vi "LoadObserverControlMatrix_zaxis.vi"(8 "NS":u16, 11 "NS_nsw":u16) -> (2 "SS FIFO TimeOut?":bool)   [LabVIEW 2017]
uses:
  fixed-point-ss/typeDefs/Bz_bram.ctl
  fixed-point-ss/typeDefs/Lz_bram.ctl
  fixed-point-ss/typeDefs/Cz_zaxis_bram.ctl
  fixed-point-ss/typeDefs/A_as_vec_bram.ctl
  <vilib>/rvi/interface/RandomDataEmulation/niFpgaRandomDataHandleErrors.vi
  <vilib>/rvi/DataTransferAndStorage/Container/Common/niFpgaContainerExecOnDevCompGetState.vi
  <vilib>/rvi/Emulation/niFpgaEmulationIsFPGAContextNoSignature.vi
  <vilib>/rvi/DataTransferAndStorage/Container/Common/niFpgaContainerGetUniqueNameForEmu.vi
  <vilib>/rvi/Emulation/niFpgaProcessEmulError.vi
  <vilib>/rvi/Emulation/niFpgaSctlEmulationGetInTimedLoop.vi
  <vilib>/rvi/errors/nirviReportUnexpectedCaseInternalError (U32).vi
  <vilib>/rvi/Memory/Memory_Emulation/niFpgaMemoryEmulationCacheClearOnFirstRun.vi
  <vilib>/rvi/Memory/Memory_Emulation/nirvimemoryEmulationManagerCache_MakeExclusive.vi
  <vilib>/rvi/Memory/Memory_Emulation/niFpgaMemoryEmulationValidateCache.vi
  <vilib>/rvi/Memory/Memory_Emulation/nirvimemoryEmulationManagerCache_InsertValue.vi
  <vilib>/Utility/error.llb/Clear Errors.vi
  <vilib>/rvi/Memory/Memory_Emulation/nirvimemoryEmulationManagerCache_ReleaseExclusive.vi
  <vilib>/rvi/Memory/Memory_Emulation/nirvimemoryEmulationManagerCache_GetValue.vi
  <vilib>/rvi/Memory/Memory_Emulation/nirvimemoryEmulationManagerCache_SetValue.vi
  <vilib>/rvi/Emulation/niFpgaSctlEmulationResourceMgr.vi
  <vilib>/rvi/DataTransferAndStorage/Container/XNode/niFpgaContainer.xnode
  <vilib>/rvi/interface/RandomDataEmulation/nirviRandomDataFpgaReadWriteTemplate.vi
  <vilib>/rvi/Memory/Memory_Emulation/niFpgaMemoryEmulationRefIn.vi
panel:
  # "NOTE: Ns is the number of states in the plant. The number of states in the \nobserver is Ns+1. Thus, for B, L, C, and A, we use NS+1. For K and Xss, we use Ns\nbecause the controller does not operate on the disturbance state, Xd."
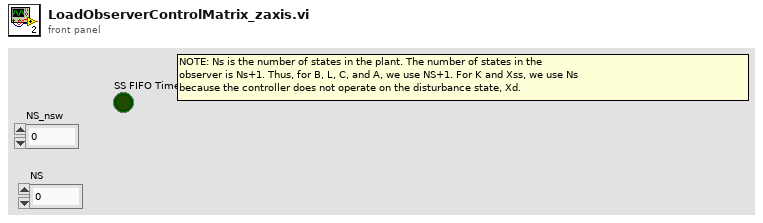
[diagram p1: front panel]
types:
  T1 = typedef "Bz_bram.ctl" = refnum<k21>
  T2 = typedef "Lz_bram.ctl" = refnum<k21>
  T3 = typedef "Cz_zaxis_bram.ctl" = refnum<k21>
  T4 = typedef "A_as_vec_bram.ctl" = refnum<k21>
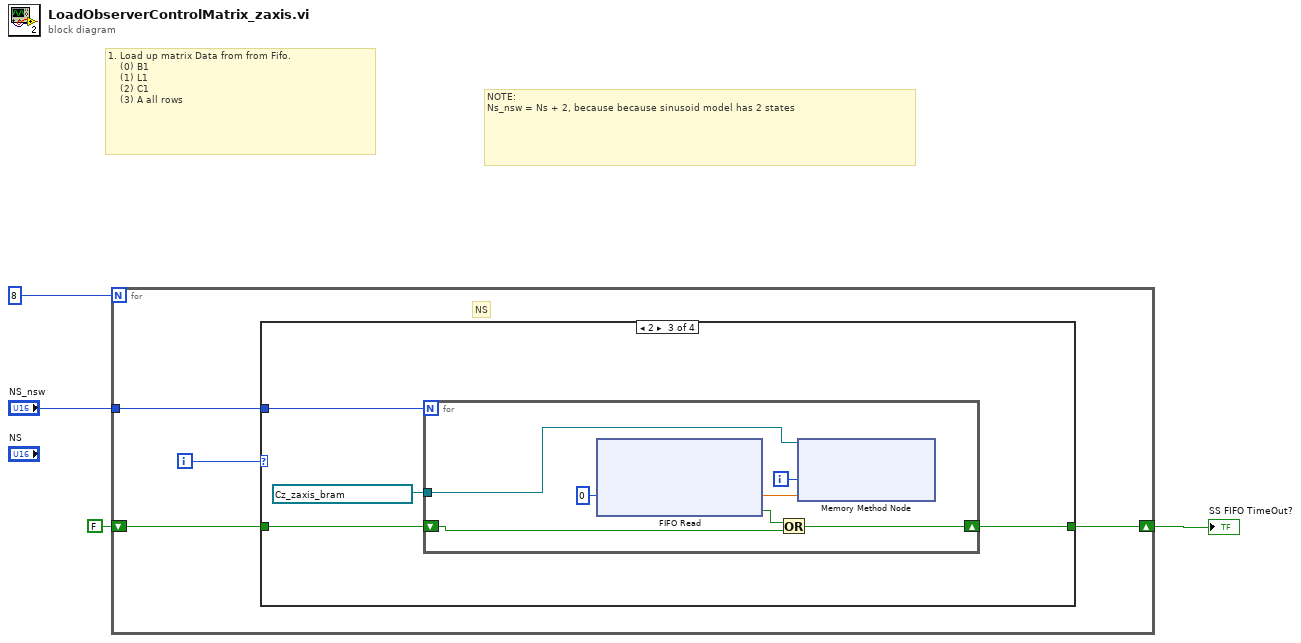
[diagram p0: block diagram]
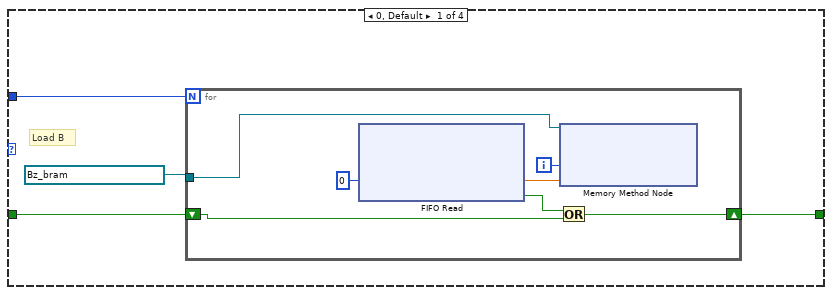
[diagram p2: hidden frame]
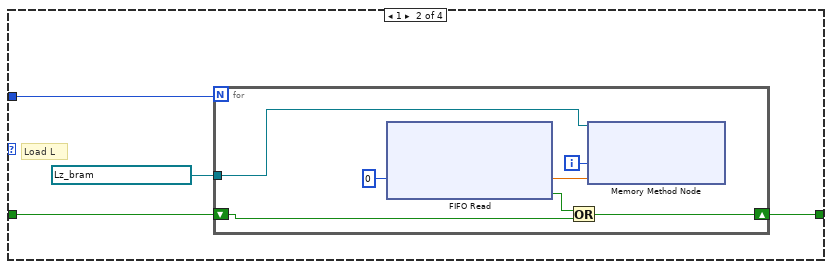
[diagram p3: hidden frame]
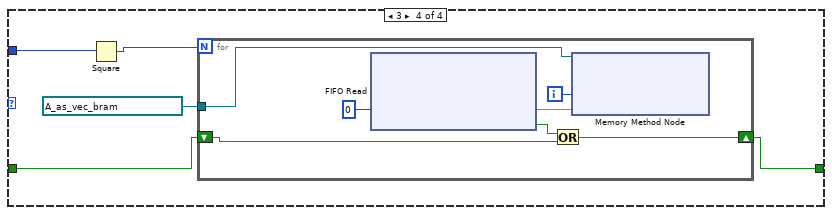
[diagram p4: hidden frame]
diagram:
  # "NOTE:\nNs_nsw = Ns + 2, because because sinusoid model has 2 states"
  # "1. Load up matrix Data from from Fifo.\n    (0) B1\n    (1) L1\n    (2) C1 \n    (3) A all rows"
  n1 = for {
    N: i16 8 -> [_]
    tunnel: "NS_nsw" -> [w7]
    shift-right: [w5] -> w2
    shift-left: FALSE -> [w6]
    i -> [w8]
    # "NS"
    n2 = case shown="2" w8 {
      tunnel: w7 -> [w12 w20 w34 w45]
      tunnel: w6 -> [w10 w22 w32 w42]
      tunnel: [w9 w21 w33 w43] -> w5
      frame 0, Default {
        # "Load B"
        n3 = for {
          N: w12 -> [_]
          tunnel: T1 "B_FXP_col1_zaxis" ("Memory") -> [w17]
          shift-right: [w14] -> w9
          shift-left: w10 -> [w13]
          i -> [w16]
          n4 = xnode ("FIFO Read")("Timeout"=i16 0) -> ("Element"=w19:sgl, "Timed Out?"=w15:bool)  [unwired: 1 in, 1 out]
          n5 = Or(x=w15, y=w13) -> (x .or. y?=w14:bool)
          n6 = xnode ("Memory Method Node")("Address"=w16, "Data"=w19, "Memory In"=w17) -> ()  [unwired: 1 out]
        }
      }
      frame 1 {
        # "Load L"
        n7 = for {
          N: w20 -> [_]
          tunnel: T2 "L_FXP_col1_zaxis" ("Memory") -> [w28]
          shift-right: [w25] -> w21
          shift-left: w22 -> [w24]
          i -> [w27]
          n8 = xnode ("FIFO Read")("Timeout"=i16 0) -> ("Element"=w30:sgl, "Timed Out?"=w26:bool)  [unwired: 1 in, 1 out]
          n9 = Or(x=w26, y=w24) -> (x .or. y?=w25:bool)
          n10 = xnode ("Memory Method Node")("Address"=w27, "Data"=w30, "Memory In"=w28) -> ()  [unwired: 1 out]
        }
      }
      frame 2 {
        n11 = for {
          N: w34 -> [_]
          tunnel: T3 "C_FXP_row1_zaxis" ("Memory") -> [w39]
          shift-right: [w36] -> w33
          shift-left: w32 -> [w35]
          i -> [w38]
          n12 = xnode ("FIFO Read")("Timeout"=i16 0) -> ("Element"=w41:sgl, "Timed Out?"=w37:bool)  [unwired: 1 in, 1 out]
          n13 = Or(x=w37, y=w35) -> (x .or. y?=w36:bool)
          n14 = xnode ("Memory Method Node")("Address"=w38, "Data"=w41, "Memory In"=w39) -> ()  [unwired: 1 out]
        }
      }
      frame 3 {
        n15 = Square(x=w45) -> (x^2=w46:u16)
        n16 = for {
          N: w46 -> [_]
          tunnel: T4 "AasCol_FXP_zaxis" ("Memory In") -> [w51]
          shift-right: [w48] -> w43
          shift-left: w42 -> [w47]
          i -> [w50]
          n17 = xnode ("FIFO Read")("Timeout"=i16 0) -> ("Element"=w53:sgl, "Timed Out?"=w49:bool)  [unwired: 1 in, 1 out]
          n18 = Or(x=w49, y=w47) -> (x .or. y?=w48:bool)
          n19 = xnode ("Memory Method Node")("Address"=w50, "Data"=w53, "Memory In"=w51) -> ()  [unwired: 1 out]
        }
      }
    }
  }
  "SS FIFO TimeOut?" <- w2
